vi "Scan from Function.vi"(0 "initial string":string, 1 "Syntax Format":T1, 11 "error in":errorcluster) -> (4 "resulting string":string, 6 "Variables Name":string[](array[string]), 8 "Variables Value":string[](array[string]), 15 "error out":errorcluster)   [LabVIEW 2016]
uses:
  Scan Syntax Format.ctl
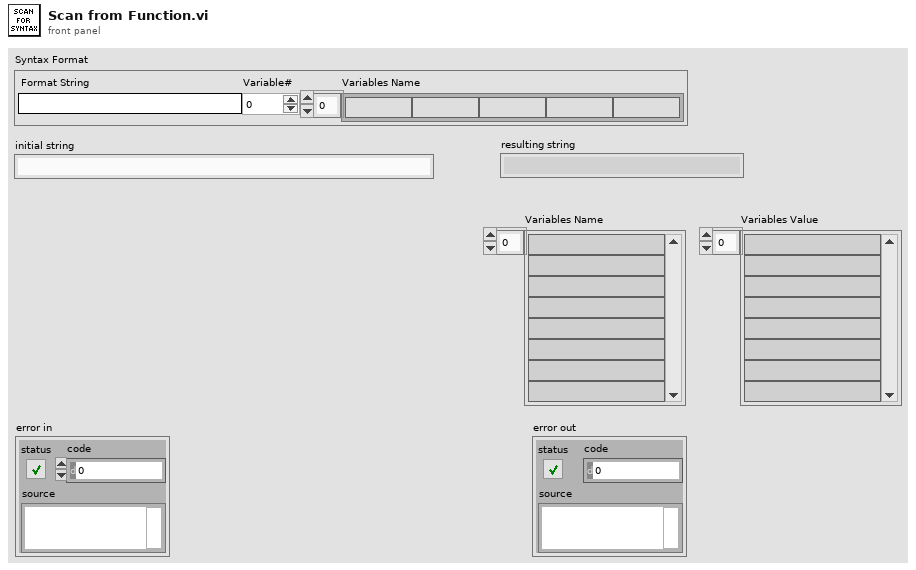
[diagram p1: front panel]
types:
  T1 = typedef "Scan Syntax Format.ctl" = cluster{"Format String":string, "Variable#":i32, "Variables Name":string[]}
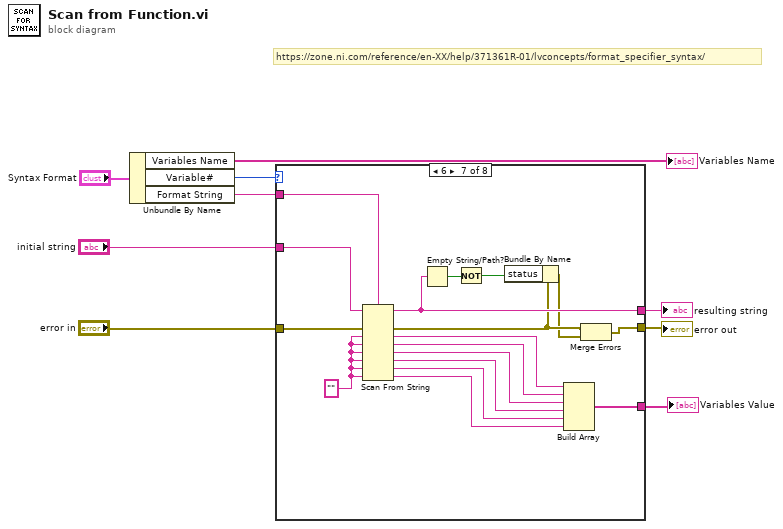
[diagram p0: block diagram]
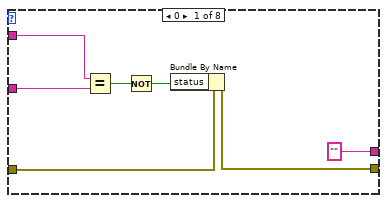
[diagram p2: hidden frame]
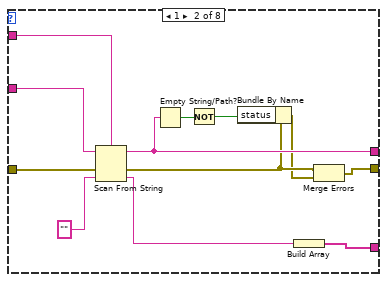
[diagram p3: hidden frame]
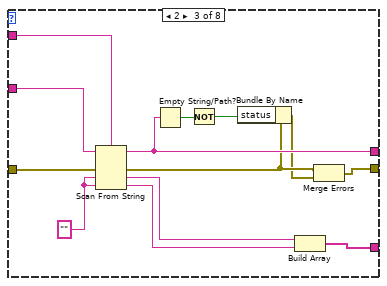
[diagram p4: hidden frame]
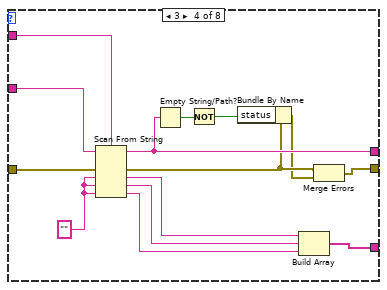
[diagram p5: hidden frame]
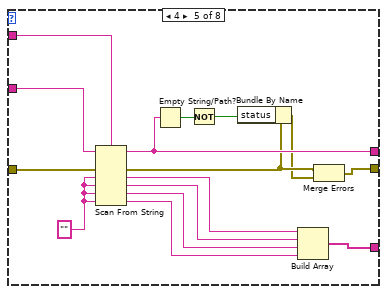
[diagram p6: hidden frame]
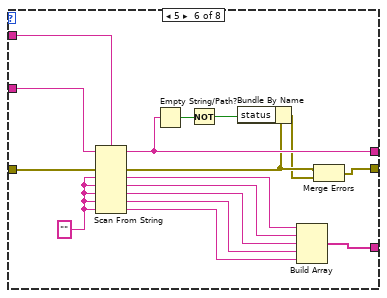
[diagram p7: hidden frame]
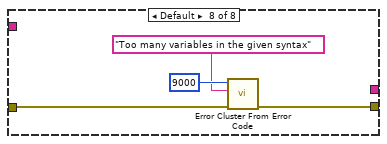
[diagram p8: hidden frame]
diagram:
  # "https://zone.ni.com/reference/en-XX/help/371361R-01/lvconcepts/format_specifier_syntax/"
  n1 = Unbundle By Name("Syntax Format") -> ("Variables Name"=→"Variables Name":string[], "Variable#"=w2:i32, "Format String"=w3:string)
  n2 = case shown="6" w2 {
    tunnel: "initial string" -> [w15 w28 w41 w55 w70 w86 w103 _]
    tunnel: "error in" -> [w13 w26 w40 w54 w69 w85 w102 w107]
    tunnel: ["" w25 w39 w53 w68 w84 w101 _] -> w7
    tunnel: [w12 w19 w33 w47 w62 w78 w95 w106] -> w5
    tunnel: w3 -> [w16 w22 w36 w50 w65 w81 w98 _]
    tunnel: [_ w17 w29 w42 w56 w71 w89 _] -> w4
    frame 0 {
      n3 = Equal?(x=w16, y=w15) -> (x = y?=w11:bool)
      n4 = Not(x=w11) -> (.not. x?=w10:bool)
      n5 = Bundle By Name(cluster=w13, "status"=w10) -> (w12:errorcluster)
    }
    frame 1 {
      n6 = Scan From String(format string=w22, input string=w28, error in=w26, default 1="") -> (remaining string=w25:string, error out=w21:errorcluster, output 1=w18:string)  [unwired: 1 in, 1 out]
      n7 = Empty String/Path?(string/path=w25) -> (empty?=w24:bool)
      n8 = Not(x=w24) -> (.not. x?=w23:bool)
      n9 = Bundle By Name(cluster=w21, "status"=w23) -> (w20:errorcluster)
      n10 = Build Array(w18) -> (w17:string[])
      n11 = Merge Errors(w21, w20) -> (w19:errorcluster)
    }
    frame 2 {
      w32 = ""
      n12 = Scan From String(format string=w36, input string=w41, error in=w40, default 1=w32, default 2=w32) -> (remaining string=w39:string, error out=w35:errorcluster, output 1=w31:string, output 2=w30:string)  [unwired: 1 in, 1 out]
      n13 = Empty String/Path?(string/path=w39) -> (empty?=w38:bool)
      n14 = Not(x=w38) -> (.not. x?=w37:bool)
      n15 = Bundle By Name(cluster=w35, "status"=w37) -> (w34:errorcluster)
      n16 = Build Array(w31, w30) -> (w29:string[])
      n17 = Merge Errors(w35, w34) -> (w33:errorcluster)
    }
    frame 3 {
      w46 = ""
      n18 = Scan From String(format string=w50, input string=w55, error in=w54, default 1=w46, default 2=w46, default 3=w46) -> (remaining string=w53:string, error out=w49:errorcluster, output 1=w45:string, output 2=w44:string, output 3=w43:string)  [unwired: 1 in, 1 out]
      n19 = Empty String/Path?(string/path=w53) -> (empty?=w52:bool)
      n20 = Not(x=w52) -> (.not. x?=w51:bool)
      n21 = Bundle By Name(cluster=w49, "status"=w51) -> (w48:errorcluster)
      n22 = Build Array(w45, w44, w43) -> (w42:string[])
      n23 = Merge Errors(w49, w48) -> (w47:errorcluster)
    }
    frame 4 {
      w61 = ""
      n24 = Scan From String(format string=w65, input string=w70, error in=w69, default 1=w61, default 2=w61, default 3=w61, default 4=w61) -> (remaining string=w68:string, error out=w64:errorcluster, output 1=w60:string, output 2=w59:string, output 3=w58:string, output 4=w57:string)  [unwired: 1 in, 1 out]
      n25 = Empty String/Path?(string/path=w68) -> (empty?=w67:bool)
      n26 = Not(x=w67) -> (.not. x?=w66:bool)
      n27 = Bundle By Name(cluster=w64, "status"=w66) -> (w63:errorcluster)
      n28 = Build Array(w60, w59, w58, w57) -> (w56:string[])
      n29 = Merge Errors(w64, w63) -> (w62:errorcluster)
    }
    frame 5 {
      w77 = ""
      n30 = Scan From String(format string=w81, input string=w86, error in=w85, default 1=w77, default 2=w77, default 3=w77, default 4=w77, default 5=w77) -> (remaining string=w84:string, error out=w80:errorcluster, output 1=w76:string, output 2=w75:string, output 3=w74:string, output 4=w73:string, output 5=w72:string)  [unwired: 1 in, 1 out]
      n31 = Empty String/Path?(string/path=w84) -> (empty?=w83:bool)
      n32 = Not(x=w83) -> (.not. x?=w82:bool)
      n33 = Bundle By Name(cluster=w80, "status"=w82) -> (w79:errorcluster)
      n34 = Build Array(w76, w75, w74, w73, w72) -> (w71:string[])
      n35 = Merge Errors(w80, w79) -> (w78:errorcluster)
    }
    frame 6 {
      w88 = ""
      n36 = Scan From String(format string=w98, input string=w103, error in=w102, default 1=w88, default 2=w88, default 3=w88, default 4=w88, default 5=w88, default 6=w88) -> (remaining string=w101:string, error out=w97:errorcluster, output 1=w94:string, output 2=w93:string, output 3=w92:string, output 4=w91:string, output 5=w90:string, output 6=w87:string)  [unwired: 1 in, 1 out]
      n37 = Empty String/Path?(string/path=w101) -> (empty?=w100:bool)
      n38 = Not(x=w100) -> (.not. x?=w99:bool)
      n39 = Bundle By Name(cluster=w97, "status"=w99) -> (w96:errorcluster)
      n40 = Build Array(w94, w93, w92, w91, w90, w87) -> (w89:string[])
      n41 = Merge Errors(w97, w96) -> (w95:errorcluster)
    }
    frame Default {
      n42 = call <vilib>:"Error Cluster From Error Code.vi"("error in (no error)"=w107, "error message (\"\")"="Too many variables in the given syntax" ("error message (\"\")"), "error code (0)"=9000) -> ("error out"=w106:errorcluster)  [unwired: 6 in]
    }
  }
  "resulting string" <- w7
  "error out" <- w5
  "Variables Value" <- w4
